vi "SetStringData.vi"(8 "error in (no error)":errorcluster caption="Fehler (Eingang, kein Fehler)", 9 "Value":string, 10 "Name":string, 11 "DictionaryString Eingang":refnum<class "DictionaryString.lvclass"> caption="DNL_LabVIEW Object in") -> (0 "error out":errorcluster caption="Fehler (Ausgang)", 3 "DictionaryString Ausgang":refnum<class "DictionaryString.lvclass"> caption="DNL_LabVIEW Object out")   [LabVIEW 2013, in "LvDictionary.lvlib" / "DictionaryString.lvclass"]
uses:
  DictionaryString.lvclass
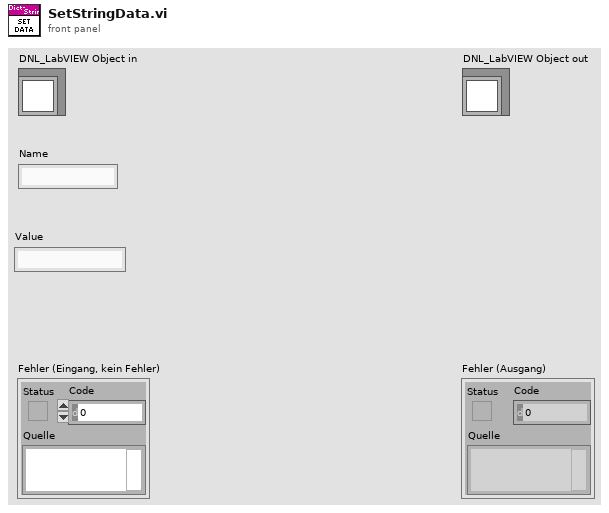
[diagram p1: front panel]
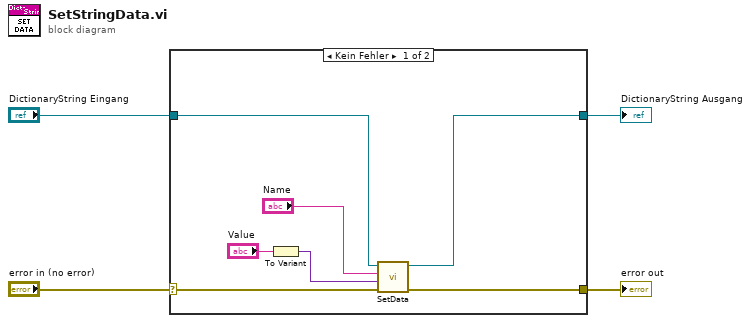
[diagram p0: block diagram]
diagram:
  n1 = case shown="Kein Fehler" "error in (no error)" {
    selector: "error in (no error)" -> [w5 w13]
    tunnel: "DictionaryString Eingang" -> [w8 w12]
    tunnel: [w7 w12] -> w2
    tunnel: [w6 w13] -> w1
    frame No Error {
      n2 = To Variant(anything="Value") -> (Variant=w9:variant)
      n3 = call-dynamic "SetData.vi"("error in (no error)"=w5, "Data"=w9, "Key"="Name", "Dictionary Eingang"=w8) -> ("error out"=w6:errorcluster, "Dictionary Ausgang"=w7:refnum<class "DictionaryString.lvclass">)  [unwired: 6 in]
    }
    frame Error {
    }
  }
  "error out" <- w1
  "DictionaryString Ausgang" <- w2
